vi "DAQmxTaskContainerAcceleratorShutter-Com-Exec.vi"(8 "error in (no error)":errorcluster, 9 "data":variant, 10 "ControlQueue":refnum<queue>, 11 "DAQmxTaksContainer_General in":refnum<class "DAQmxTaksContainer_General.lvclass">) -> (0 "error out":errorcluster, 3 "DAQmxTaksContainer_General out":refnum<class "DAQmxTaksContainer_General.lvclass">)   [LabVIEW 2015, in "DAQmxTaksContainer_General.lvclass"]
uses:
  DAQmxTaksContainer_General.lvclass
  dependecies/ControlsVIs/Clusters-def/ProtypeCommand-DAQmxReply.ctl
  dependecies/ControlsVIs/Clusters-def/SERVER-Commands.ctl
  DAQmxTask.lvclass
  Control/Control-Server/Control-Server.lvclass
panel:
  out "DAQmxTaskContainer_General out":refnum<class "DAQmxTaksContainer_General.lvclass">
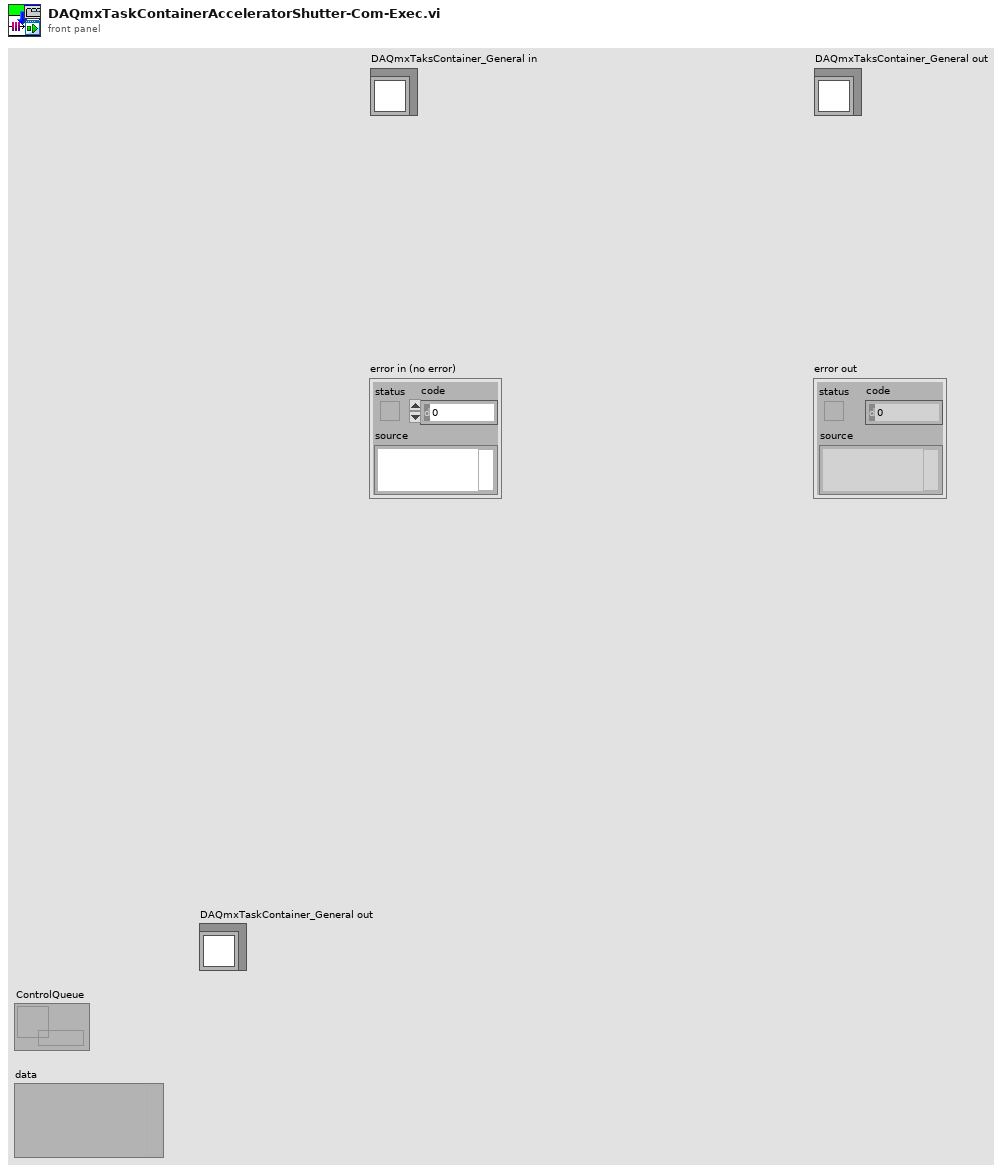
[diagram p1: front panel]
types:
  T1 = typedef "Control-Server.lvclass/SERVER-Commands.ctl" = string
  T2 = typedef "ProtypeCommand-DAQmxReply.ctl" = cluster{"On/Off":bool, "error out":errorcluster}
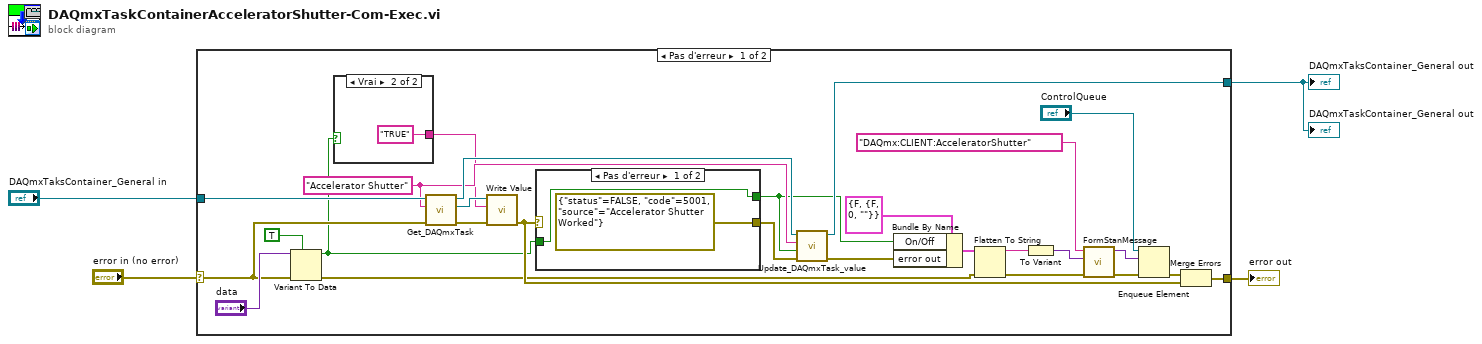
[diagram p0: block diagram]
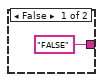
[diagram p2: hidden frame]
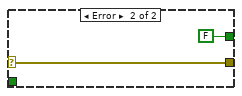
[diagram p3: hidden frame]
diagram:
  n1 = case shown="Pas d'erreur" "error in (no error)" {
    selector: "error in (no error)" -> [w27 w39]
    tunnel: [w8 w38] -> w4
    tunnel: "DAQmxTaksContainer_General in" -> [w30 w38]
    tunnel: [w29 w39] -> w3
    frame No Error {
      w7 = "Accelerator Shutter" ("Task name")
      n2 = Variant To Data(error in=w27, type=TRUE, Variant="data") -> (data=w21:bool, error out=w18:errorcluster)
      n3 = case shown="Vrai" w21 {
        tunnel: ["FALSE" ("Data") "TRUE" ("Data")] -> w5
        frame False {
        }
        frame True {
        }
      }
      n4 = call "Get_DAQmxTask.vi"("error in (no error)"=w27, "Task name"=w7, "DAQmxTaksContainer_General in"=w30) -> ("error out"=w26:errorcluster, "DAQmx Task"=w24:refnum<class "DAQmxTask.lvclass">, "DAQmxTaksContainer_General out"=w9:refnum<class "DAQmxTaksContainer_General.lvclass">)  [unwired: 6 in]
      n5 = call-dynamic "Write Value.vi"("error in (no error)"=w26, "Data"=w5, "DAQmxTask en entrée"=w24) -> ("error out"=w23:errorcluster)  [unwired: 7 in, 1 out]
      n6 = case shown="Pas d'erreur" w23 {
        selector: w23 -> [_ w37]
        tunnel: [errorcluster {"status"=FALSE, "code"=5001, "source"="Accelerator Shutter Worked"} ("error constant") w37] -> w11
        tunnel: [w34 FALSE] -> w6
        tunnel: w21 -> [w34 _]
        frame No Error {
        }
        frame Error {
        }
      }
      n7 = call "Update_DAQmxTask_value.vi"("error in (no error)"=w11, "Value"=w6, "Task name"=w7, "DAQmxTaksContainer_General in"=w9) -> ("error out"=w10:errorcluster, "DAQmxTaksContainer_General out"=w8:refnum<class "DAQmxTaksContainer_General.lvclass">)  [unwired: 6 in]
      n8 = Bundle By Name(cluster=T2 {"On/Off"=FALSE, "error out"={"status"=FALSE, "code"=0, "source"=""}} ("output cluster"), "On/Off"=w6, "error out"=w10) -> (w19:T2)
      n9 = Flatten To String(anything=w19, error in (no error)=w18) -> (data string=w20:string, error out=w15:errorcluster)  [unwired: 2 in, 1 out]
      n10 = To Variant(anything=w20) -> (Variant=w16:variant)
      n11 = call "FormStanMessage.vi"("error in"=w15, "data"=w16, "Command"=T1 "DAQmx:CLIENT:AcceleratorShutter" ("Commands")) -> ("error out"=w13:errorcluster, "message"=w12:variant)  [unwired: 7 in]
      n12 = Enqueue Element(queue="ControlQueue", element=w12, error in (no error)=w13) -> (error out=w17:errorcluster)  [unwired: 1 in, 2 out]
      n13 = Merge Errors(w17, w23) -> (w29:errorcluster)
    }
    frame Error {
    }
  }
  "error out" <- w3
  "DAQmxTaksContainer_General out" <- w4
  "DAQmxTaskContainer_General out" <- w4
